vi "WPI_IMU_ADIS16448 Read Register Array.vi"(8 "error in":errorcluster, 10 "Registers":u8[](array[numeric]), 11 "SPI Ref":T1) -> (0 "error out":errorcluster, 2 "Data":u16[](array[numeric]), 3 "SPIDevRef":T1)   [LabVIEW 2014, in "ADIS16448.lvlib"]
uses:
  ADIS16448.lvlib
  <vilib>/Rock Robotics/WPI/SPI/WPI_SPIDevRef.ctl
  <vilib>/Rock Robotics/SystemInterfaces/Typedef/FPGA_TypedefDigitalModule.ctl
  <vilib>/Rock Robotics/SystemInterfaces/spilib/spi_bus.ctl
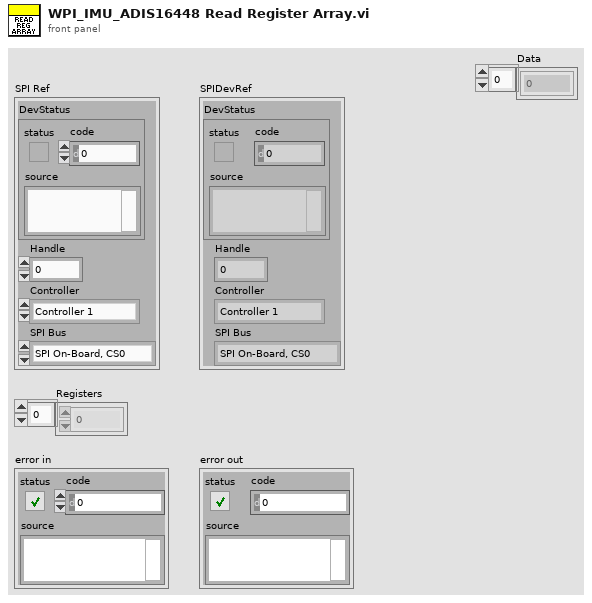
[diagram p1: front panel]
types:
  T1 = typedef "WPI_SPIDevRef.ctl" = cluster{"DevStatus":errorcluster, "Handle":i32, "Controller":T2, "SPI Bus":T3}
  T2 = typedef "FPGA_TypedefDigitalModule.ctl" = enum16{"Controller 1"}
  T3 = typedef "spi_bus.ctl" = enum16{"SPI On-Board, CS0", "SPI On-Board, CS1", "SPI On-Board, CS2", "SPI On-Board, CS3", "SPI MXP", "Invalid"}
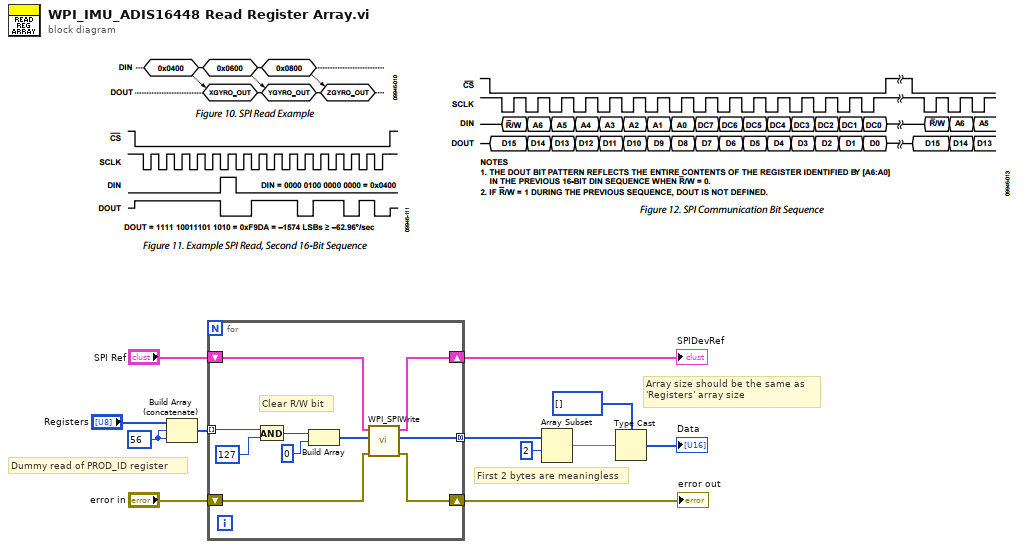
[diagram p0: block diagram]
diagram:
  w1 = u8 56 ("new element/subarray")
  # "Dummy read of PROD_ID register"
  # "Array size should be the same as \n'Registers' array size"
  # "First 2 bytes are meaningless"
  n1 = Build Array (concatenate)("Registers", w1, w1) -> (w2:u8[])
  n2 = for {
    shift-right: [w16] -> w5
    shift-left: "SPI Ref" -> [w18]
    shift-right: [w15] -> w6
    shift-left: "error in" -> [w17]
    tunnel: [w13] -> w4 mode=concatenating
    tunnel: w2 -> [w14] mode=indexing
    # "Clear R/W bit"
    n3 = And(x=w14, y=u8 127) -> (x .and. y?=w20:u8)
    n4 = Build Array(w20, u8 0) -> (w19:u8[])
    n5 = call <vilib>:"WPI_SPIWrite.vi"("error in (no error)"=w17, "Data To Send"=w19, "SPIDevRef"=w18) -> ("error out"=w15:errorcluster, "Received Data"=w13:u8[], "SPIDevRef"=w16:T1)  [unwired: 6 in]
  }
  "SPIDevRef" <- w5
  "error out" <- w6
  n6 = Array Subset(array=w4, index=2) -> (w9:u8[])  [unwired: 1 in]
  n7 = Type Cast(type=u16[] [], x=w9) -> (*(type *) &x=→"Data":u16[])
